vi "同步D触发器（下降沿触发）.vi"(4 "CP":bool, 7 "D":bool) -> (3 "Q":bool)   [LabVIEW 2012, in "触发器.lvlib"]
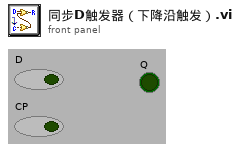
[diagram p1: front panel]
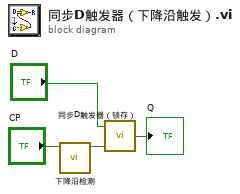
[diagram p0: block diagram]
diagram:
  n1 = call "下降沿检测.vi"("input"="CP") -> ("output"=w2:bool)  [unwired: 9 in, 1 out]
  n2 = call "同步D触发器（锁存）.vi"("CP"=w2, "D"="D") -> ("Q"=→"Q":bool)  [unwired: 1 in]
